vi "PH_gentec_M-Link.set Data Flow.vi"(0 "i ref in":refnum<vi>, 2 "VISA resource in":refnum<visa-resource-name>, 5 "error in":errorcluster) -> (11 "Timeout":bool, 13 "Data read":string[](array[string]), 14 "i ref out":refnum<vi>, 16 "VISA resource out":refnum<visa-resource-name>, 17 "Error":bool, 18 "Failure":bool, 19 "error out":errorcluster)   [LabVIEW 2014, in "PH_gentec_M-Link.lvlib"]
doc: "This VI writes wanted Settings to the Device and checks the result."
uses:
  PH_gentec_M-Link.lvlib
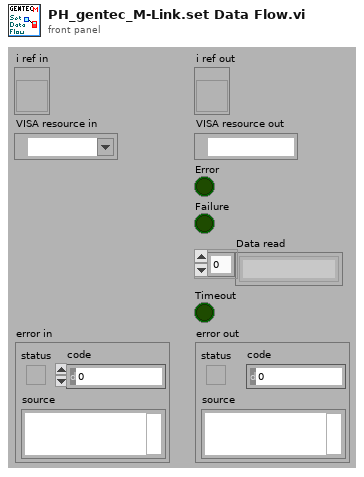
[diagram p1: front panel]
types:
  T1 = typedef "PH_gentec_M-Link.lvlib/PH_gentec_M-Link.i attribute.ctl" = cluster{"GUI References":cluster{"Wanted Head Settings":refnum<vi>, "Current Head Settings":refnum<vi>, "Set Auto Range":refnum<vi>, "Trigger Polarity":refnum<vi>, "Trigger Source":refnum<vi>, "Waveform Averages":refnum<vi>, "Continuous":refnum<vi>, "get one Value":refnum<vi>}, "Wanted Head Settings":T2, "Current Head Settings":T2}
  T2 = typedef "PH_gentec_M-Link.lvlib/PH_gentec_M-Link.Head Settings.ctl" = cluster{"Measurement Mode":T3, "Enable Anticipation":bool, "Set Auto Range":bool, "Block Signal":bool, "Set Head Attenuator":bool, "Enable SSE":bool, "Trigger Polarity":T4, "Trigger Source":T5, "Waveform Averages":T6, "Set Zero":i32, "Current":i32, "Start Data Flow":bool}
  T3 = typedef "gentec-M-Link - Driver.lvlib/gentec-M-Link.Measurement Mode.ctl" = u16
  T4 = typedef "gentec-M-Link - Driver.lvlib/gentec-M-Link.Trigger Polarity.ctl" = u16
  T5 = typedef "gentec-M-Link - Driver.lvlib/gentec-M-Link.Trigger Source.ctl" = u16
  T6 = typedef "gentec-M-Link - Driver.lvlib/gentec-M-Link.Waveform Averages.ctl" = u16
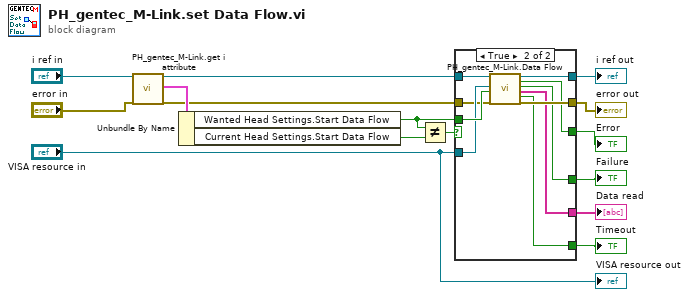
[diagram p0: block diagram]
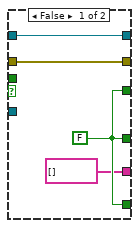
[diagram p2: hidden frame]
diagram:
  n1 = call "PH_gentec_M-Link.get i attribute.vi"("i ref in"="i ref in", "error in (no error)"="error in") -> ("i ref out"=w8:refnum<vi>, "i attribute"=w11:T1, "error out"=w10:errorcluster)  [unwired: 15 in]
  n2 = Unbundle By Name(w11) -> ("Wanted Head Settings.Start Data Flow"=w13:bool, "Current Head Settings.Start Data Flow"=w12:bool)
  n3 = Not Equal?(x=w13, y=w12) -> (x != y?=w1:bool)
  n4 = case shown="True" w1 {
    tunnel: [w16 w24] -> w15
    tunnel: [w17 w26] -> w14
    tunnel: w13 -> [_ w29]
    tunnel: w10 -> [w16 w25]
    tunnel: w8 -> [w17 w27]
    tunnel: "VISA resource in" -> [_ w28]
    tunnel: [w19 w23] -> w5
    tunnel: [w19 w22] -> w4
    tunnel: [w19 w20] -> w3
    tunnel: [string[] [] w21] -> w2
    frame False {
      w19 = FALSE
    }
    frame True {
      n5 = call "PH_gentec_M-Link.Data Flow.vi"("i ref in"=w27, "VISA resource in"=w28, "Data Flow State to set"=w29, "error in"=w25) -> ("i ref out"=w26:refnum<vi>, "Error"=w23:bool, "Failure"=w22:bool, "Data Read"=w21:string[], "Read Timeout"=w20:bool, "error out"=w24:errorcluster)  [unwired: 10 in]
    }
  }
  "error out" <- w15
  "i ref out" <- w14
  "Error" <- w5
  "Failure" <- w4
  "Timeout" <- w3
  "Data read" <- w2
  "VISA resource out" <- "VISA resource in"
